vi "svx_PlotWaterfallPlots.vi"(0 "Dec/Cropped in":T1={"Dec/Cropped in"={"z0"=0.0, "dz"=1.0, "Plots"=[]}, "Lines"=[]}, 3 "XYGraph in":refnum<vi>, 5 "Z Scale Graph ref":refnum<vi>, 8 "Cropped Info in":cluster{"First Index":i32, "Length":i32}, 9 "Data In":T2, 11 "State Out":T4={"X Scale Width %"=50.0, "Y Scale Height %"=50.0, "X-Axis Range"={"Minimum"=0.0, "Maximum"=10.0}, "Y-Axis Range"={"Minimum"=0.0, "Maximum"=10.0}, "Z-Axis Range"={"Minimum"=0.0, "Maximum"=10.0}, "Plot Color"=61212, "Frame Color"=16252785, "Background Color"=16777222, "Initial AutoScale Y"=TRUE, "AutoScale X"=2, "AutoScale Y"=2, "AutoScale Z"=2, "Plot Transparency"=FALSE, "X-Axis Name"="Frequency", "Y-Axis Name"="Amplitude", "Z-Axis Name"="", "X-Axis Scaling Factor"={"Offset"=0.0, "Multiplier"=1.0}, "Y-Axis Scaling Factor"={"Offset"=0.0, "Multiplier"=1.0}, "Z-Axis Scaling Factor"={"Offset"=0.0, "Multiplier"=1.0}, "X-Scale Visible"=TRUE, "Y-Scale Visible"=TRUE, "Z-Scale Visible"=TRUE, "X-Scale Label Visible"=TRUE, "Y-Scale Label Visible"=TRUE, "Z-Scale Label Visible"=TRUE, "X-Axis Range Scaled"={"Minimum"=0.0, "Maximum"=10.0}, "Y-Axis Range Scaled"={"Minimum"=0.0, "Maximum"=10.0}, "Z-Axis Range Scaled"={"Minimum"=0.0, "Maximum"=10.0}, "Rev Z Order"=FALSE, "X-Scale Format Str"="%#.4g", "Y-Scale Format Str"="%#.4g", "Z-Scale Format Str"="%#.4g", "Decor color"=12369084, "Scale Range Change"=refnum, "out of state queue"=refnum, "property nodes"=refnum, "Lines"=[], "Line Properties"={"Line Color"=61212, "Line Width"=61212, "Line Style"=enum."Dash", "DisplayLines"=FALSE}} caption="State" {"Line Properties"."Line Width" min=1}) -> ()   [LabVIEW 2017, in "SVX Waterfall Graph.xctl"]
uses:
  <vilib>/addons/_XControls/Waterfall Graph/SVX Waterfall Graph.xctl
  <vilib>/addons/_XControls/Waterfall Graph/subVIs/svx_Waterfall State.ctl
  <vilib>/addons/_NISVFA/_Shared subVIs/Controls/svc_Cluster of Array of Cluster of XYZ.ctl
  <vilib>/addons/_XControls/Waterfall Graph/subVIs/svx_Waterfall Data.ctl
  <vilib>/addons/_XControls/Waterfall Graph/subVIs/svx_CroppedData.ctl
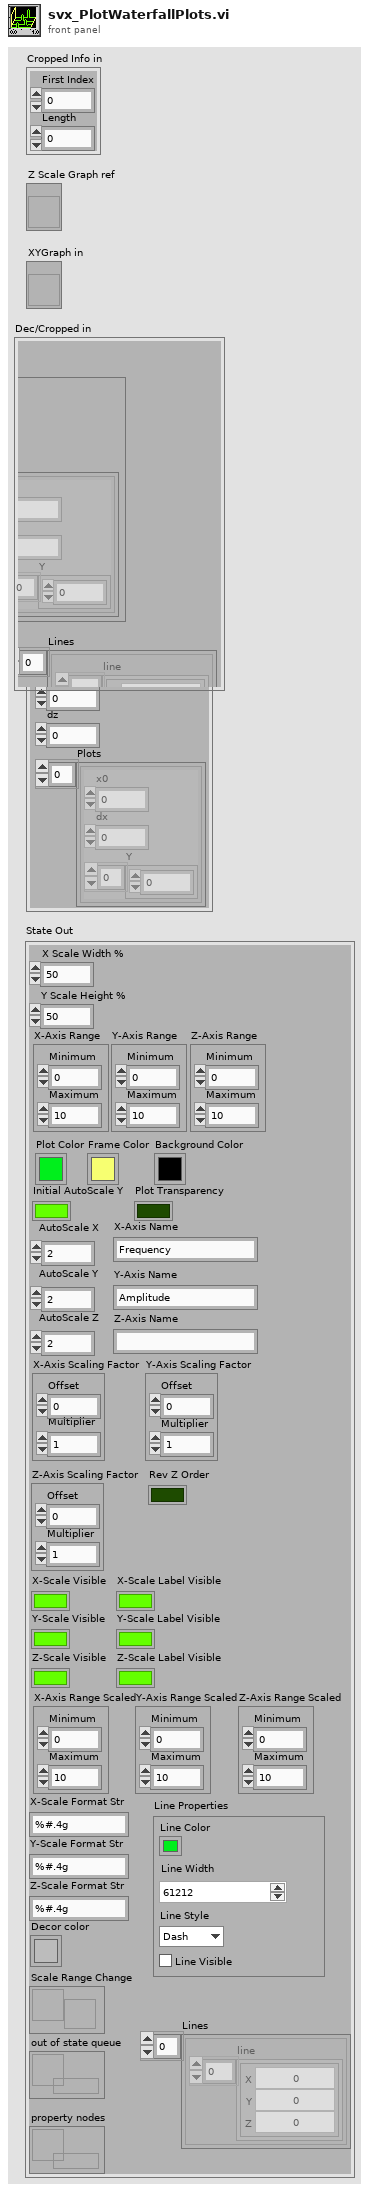
[diagram p1: front panel]
types:
  T1 = typedef "SVX Waterfall Graph.xctl/svx_CroppedData.ctl" = cluster{"Dec/Cropped in":T2, "Lines":T3[]}
  T2 = typedef "SVX Waterfall Graph.xctl/svx_Waterfall Data.ctl" = cluster{"z0":dbl, "dz":dbl, "Plots":cluster{"x0":dbl, "dx":dbl, "Y":dbl[]}[]}
  T3 = typedef "svc_Cluster of Array of Cluster of XYZ.ctl" = cluster{"line":cluster{"X":dbl, "Y":dbl, "Z":dbl}[]}
  T4 = typedef "SVX Waterfall Graph.xctl/svx_Waterfall State.ctl" = cluster{"X Scale Width %":dbl, "Y Scale Height %":dbl, "X-Axis Range":cluster{"Minimum":dbl, "Maximum":dbl}, "Y-Axis Range":cluster{"Minimum":dbl, "Maximum":dbl}, "Z-Axis Range":cluster{"Minimum":dbl, "Maximum":dbl}, "Plot Color":u32, "Frame Color":u32, "Background Color":u32, "Initial AutoScale Y":bool, "AutoScale X":u8, "AutoScale Y":u8, "AutoScale Z":u8, "Plot Transparency":bool, "X-Axis Name":string, "Y-Axis Name":string, "Z-Axis Name":string, "X-Axis Scaling Factor":cluster{"Offset":dbl, "Multiplier":dbl}, "Y-Axis Scaling Factor":cluster{"Offset":dbl, "Multiplier":dbl}, "Z-Axis Scaling Factor":cluster{"Offset":dbl, "Multiplier":dbl}, "X-Scale Visible":bool, "Y-Scale Visible":bool, "Z-Scale Visible":bool, "X-Scale Label Visible":bool, "Y-Scale Label Visible":bool, "Z-Scale Label Visible":bool, "X-Axis Range Scaled":cluster{"Minimum":dbl, "Maximum":dbl}, "Y-Axis Range Scaled":cluster{"Minimum":dbl, "Maximum":dbl}, "Z-Axis Range Scaled":cluster{"Minimum":dbl, "Maximum":dbl}, "Rev Z Order":bool, "X-Scale Format Str":string, "Y-Scale Format Str":string, "Z-Scale Format Str":string, "Decor color":u32, "Scale Range Change":refnum<user-event>, "out of state queue":refnum<queue>, "property nodes":refnum<queue>, "Lines":T3[], "Line Properties":cluster{"Line Color":u32, "Line Width":u16, "Line Style":enum32{"Solid", "Dash", "Dot", "DashDot", "DashDotDot"}, "DisplayLines":bool}}
  T5 = enum32{"Solid", "Dash", "Dot", "DashDot", "DashDotDot"}
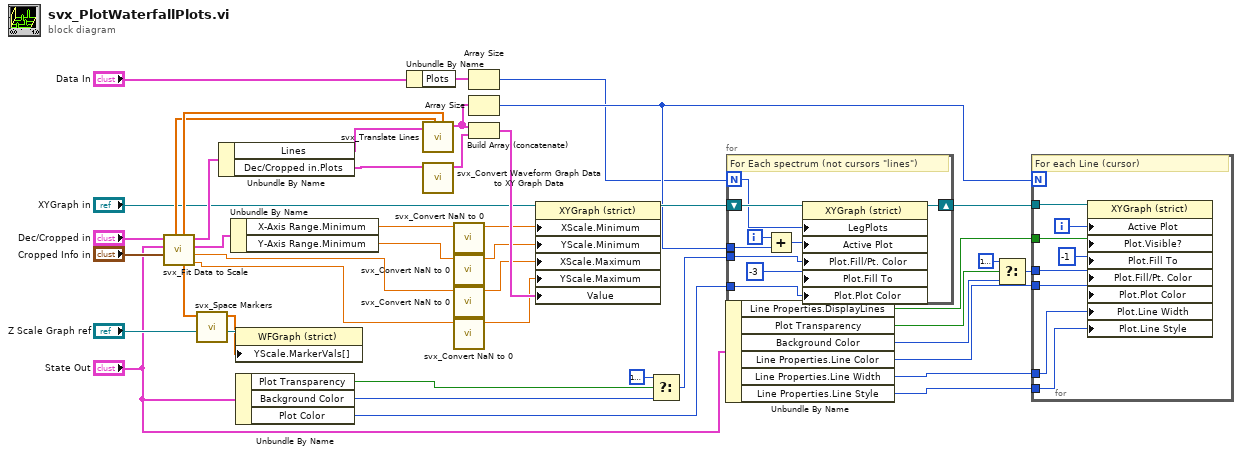
[diagram p0: block diagram]
diagram:
  n1 = call <vilib>:"svx_Fit Data to Scale.vi"("Cropped Info"="Cropped Info in", "Display State In"="State Out", "Data In"="Dec/Cropped in") -> ("Waveform YScale Max"=w4:dbl, "Waveform XScale Max"=w5:dbl, "Display State Out"=w30:T4, "Data Out"=w31:T1, "Markers"=w36:dbl[], "Y Offset Per spectrum"=w42:dbl[], "Xoffset per spectrum"=w41:dbl[])  [unwired: 2 in]
  n2 = call <vilib>:"svx_Space Markers.vi"("Z Scale Graph ref"="Z Scale Graph ref", "markers in"=w36) -> ("Z Scale Graph ref out"=w39:refnum<vi>, "markers out"=w37:dbl[])  [unwired: 8 in]
  n3 = Unbundle By Name(w31) -> ("Lines"=w9:T3[], "Dec/Cropped in.Plots"=w40:cluster{"x0":dbl, "dx":dbl, "Y":dbl[]}[])
  n4 = Unbundle By Name(w30) -> ("X-Axis Range.Minimum"=w8:dbl, "Y-Axis Range.Minimum"=w6:dbl)
  n5 = property on="Property Node" class="WFGraph (strict)"(reference=w39, "YScale.MarkerVals[]"=w37) -> ()  [unwired: 1 in, 2 out]
  n6 = Unbundle By Name("State Out") -> ("Plot Transparency"=w18:bool, "Background Color"=w19:u32, "Plot Color"=w29:u32)
  n7 = Unbundle By Name("Data In") -> ("Plots"=w34:cluster{"x0":dbl, "dx":dbl, "Y":dbl[]}[])
  n8 = call <vilib>:"svx_Translate Lines.vi"("Y Offset Per spectrum"=w42, "Xoffset per spectrum"=w41, "Lines"=w9) -> ("Lines XY Plots"=w28:cluster{"X":dbl[], "Y":dbl[]}[])  [unwired: 8 in]
  n9 = call <vilib>:"svx_Convert Waveform Graph Data to XY Graph Data.vi"("Waveform Graph"=w40) -> ("XY Graph"=w43:cluster{"X":dbl[], "Y":dbl[]}[])  [unwired: 10 in]
  n10 = call <vilib>:"svx_Convert NaN to 0.vi"("Double"=w8) -> ("Converted Value"=w7:dbl)  [unwired: 10 in]
  n11 = call <vilib>:"svx_Convert NaN to 0.vi"("Double"=w6) -> ("Converted Value"=w3:dbl)  [unwired: 10 in]
  n12 = call <vilib>:"svx_Convert NaN to 0.vi"("Double"=w5) -> ("Converted Value"=w2:dbl)  [unwired: 10 in]
  n13 = call <vilib>:"svx_Convert NaN to 0.vi"("Double"=w4) -> ("Converted Value"=w1:dbl)  [unwired: 10 in]
  n14 = Array Size(array=w34) -> (size(s)=w21:i32)
  n15 = Array Size(array=w28) -> (size(s)=w22:i32)
  n16 = Build Array (concatenate)(w28, w43) -> (w44:cluster{"X":dbl[], "Y":dbl[]}[])
  n17 = property on="Property Node" class="XYGraph (strict)"(reference="XYGraph in", "XScale.Minimum"=w7, "YScale.Minimum"=w3, "XScale.Maximum"=w2, "YScale.Maximum"=w1, "Value"=w44) -> (reference out=w25:refnum<vi>)  [unwired: 1 in, 1 out]
  n18 = Select(t=u32 16777216, s=w18, f=w19) -> (s? t:f=w23:u32)
  n19 = Unbundle By Name("State Out") -> ("Line Properties.DisplayLines"=w17:bool, "Plot Transparency"=w11:bool, "Background Color"=w12:u32, "Line Properties.Line Color"=w16:u32, "Line Properties.Line Width"=w15:u16, "Line Properties.Line Style"=w14:T5)
  n20 = for {
    N: w21 -> [w45]
    tunnel: w29 -> [w53]
    tunnel: w22 -> [w52]
    tunnel: w23 -> [w48]
    shift-right: [w47] -> w27
    shift-left: w25 -> [w46]
    i -> [w51]
    # "For Each spectrum (not cursors \"lines\")"
    n21 = Add(x=w51, y=w52) -> (x+y=w50:i32)
    n22 = property on="Property Node" class="XYGraph (strict)"(reference=w46, "LegPlots"=w45, "Active Plot"=w50, "Plot.Fill/Pt. Color"=w48, "Plot.Fill To"=i16 -3, "Plot.Plot Color"=w53) -> (reference out=w47:refnum<vi>)  [unwired: 1 in, 1 out]
  }
  n23 = Select(t=u32 16777216, s=w11, f=w12) -> (s? t:f=w10:u32)
  n24 = for {
    N: w22 -> [_]
    tunnel: w27 -> [w61]
    tunnel: w17 -> [w58]
    tunnel: w16 -> [w57]
    tunnel: w15 -> [w56]
    tunnel: w14 -> [w55]
    tunnel: w10 -> [w54]
    i -> [w59]
    # "For each Line (cursor)"
    n25 = property on="Property Node" class="XYGraph (strict)"(reference=w61, "Active Plot"=w59, "Plot.Visible?"=w58, "Plot.Fill To"=i16 -1, "Plot.Fill/Pt. Color"=w54, "Plot.Plot Color"=w57, "Plot.Line Width"=w56, "Plot.Line Style"=w55) -> ()  [unwired: 1 in, 2 out]
  }
